vi "Module Type.vi"(11 "Config Alert Module in":refnum<class "Config Monitor Module.lvclass">) -> (2 "Module Type":string)   [LabVIEW 2020, in "VolatusGUI.lvlib" / "Config Monitor Module.lvclass"]
uses:
  Config Monitor Module.lvclass
  Config Monitor Module.lvclass/Config Monitor Module.ctl
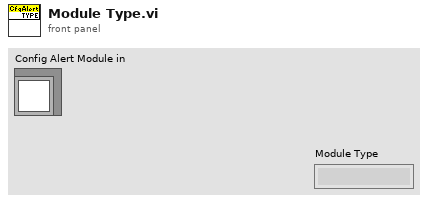
[diagram p1: front panel]
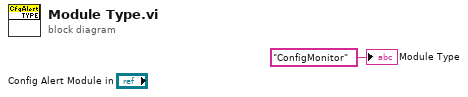
[diagram p0: block diagram]
diagram:
  "Module Type" <- "ConfigMonitor" ("Module Type")
